vi "Write Sudoku Int.vi"(8 "error in (no error)":errorcluster, 10 "Sudoku Int":u8[][](array[numeric]), 11 "Sudoku Class in":refnum<class "Sudoku Class.lvclass">) -> (0 "error out":errorcluster, 3 "Sudoku Class out":refnum<class "Sudoku Class.lvclass">)   [LabVIEW 2015, in "Sudoku Library.lvlib" / "Sudoku Class.lvclass"]
doc: "Created IvanLis by LabVIEW Portal\nProfile: http://labviewportal.org/memberlist.php?mode=viewprofile&u=987\neMail: IvanLisanov@gMail.com\nTelegram: https://t.me/IvanLis"
uses:
  Sudoku Class.lvclass
  Sudoku Class.lvclass/Sudoku Class.ctl
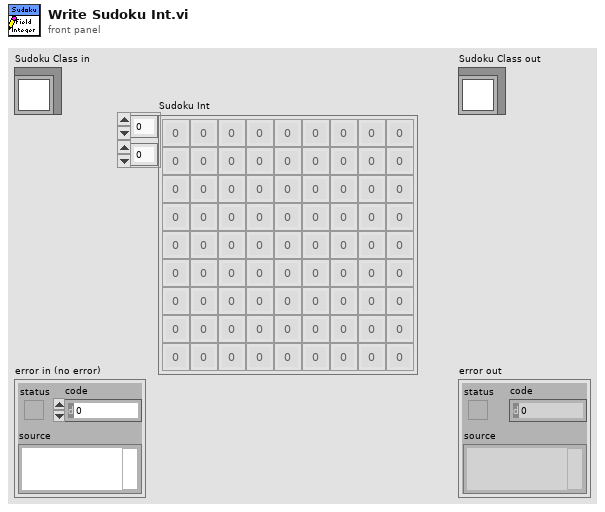
[diagram p1: front panel]
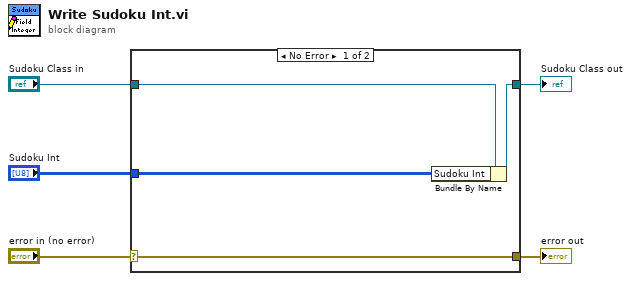
[diagram p0: block diagram]
diagram:
  n1 = case shown="No Error" "error in (no error)" {
    selector: "error in (no error)" -> [w9 w10]
    tunnel: [w9 w10] -> w4
    tunnel: [w7 w11] -> w2
    tunnel: "Sudoku Class in" -> [w8 w11]
    tunnel: "Sudoku Int" -> [w6 _]
    frame No Error {
      n2 = Bundle By Name(cluster=w8, "Sudoku Int"=w6) -> (w7:refnum<class "Sudoku Class.lvclass">)
    }
    frame Error {
    }
  }
  "error out" <- w4
  "Sudoku Class out" <- w2
